vi "GT Set Profile Config.vi"(8 "error in (no error)":errorcluster caption="错误输入（无错误）", 9 "pProfile":T1, 10 "profile":i16, 11 "cardNum":i16) -> (0 "error out":errorcluster caption="错误输出", 1 "pProfile out":T1, 3 "function return":i16)   [LabVIEW 2020, in "gts1.lvlib"]
doc: "GT_API GT_SetProfileConfig(short cardNum,short profile,TProfileConfig *pProfile);"
uses:
  gts1.lvlib
  dll/32bit/multi_card/gts.dll
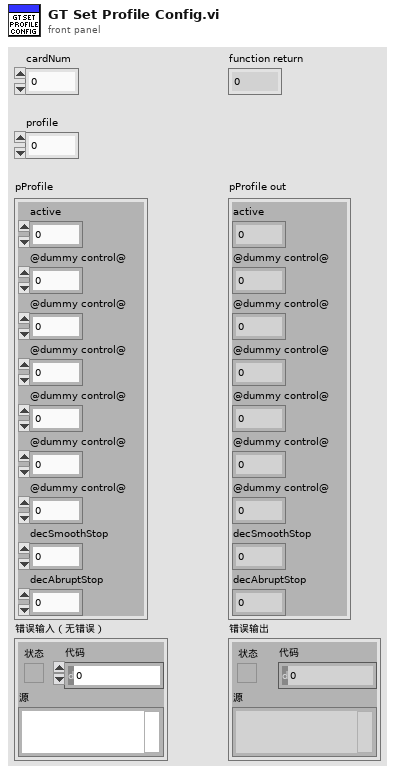
[diagram p1: front panel]
types:
  T1 = cluster{"active":i16, "@dummy control@":i8, "@dummy control@":i8, "@dummy control@":i8, "@dummy control@":i8, "@dummy control@":i8, "@dummy control@":i8, "decSmoothStop":dbl, "decAbruptStop":dbl}
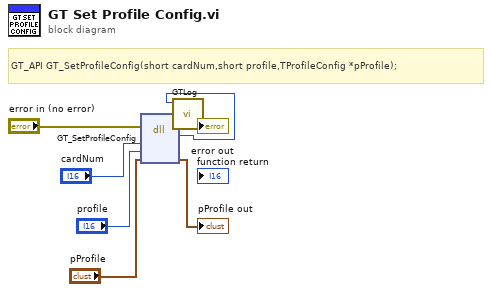
[diagram p0: block diagram]
diagram:
  # "GT_API GT_SetProfileConfig(short cardNum,short profile,TProfileConfig *pProfile);"
  n1 = dll-call lib="C:/1228/dll/32bit/multi_card/gts.dll" fn="GT_SetProfileConfig"(error in="error in (no error)", "cardNum"="cardNum", "profile"="profile", "pProfile"="pProfile") -> (error out=w3:errorcluster, w1:i16, "pProfile"=→"pProfile out":T1)  [unwired: 4 in, 1 out]
  n2 = call "GTLog.vi"("error in (no error)"=w3, "Numeric"=w1) -> ("error out"=→"error out":errorcluster)  [unwired: 9 in]
